vi "4.2.4.vi"() -> ()   [LabVIEW 2017]
panel:
  in  "stop":bool
  in  "Frequency 2":dbl
  in  "Frequency 1":dbl
  in  "Phase 2":dbl
  in  "Phase 1":dbl
  out "XY Graph":cluster{"X":dbl[], "Y":dbl[]}[](graph)
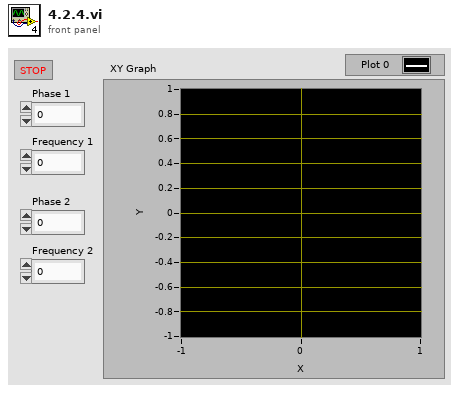
[diagram p1: front panel]
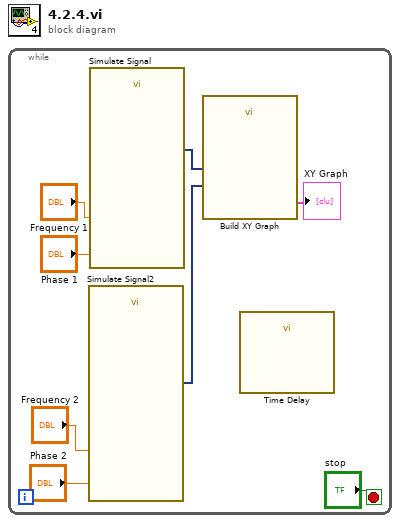
[diagram p0: block diagram]
diagram:
  n1 = while {
    stop <- "stop" stop-if-true
    n2 = call "Simulate Signal2"("Frequency"="Frequency 2", "Phase"="Phase 2") -> ("Sine"=w7:dynamicdata)  [unwired: 12 in, 1 out]
    n3 = call "Simulate Signal"("Frequency"="Frequency 1", "Phase"="Phase 1") -> ("Sine"=w8:dynamicdata)  [unwired: 12 in, 1 out]
    n4 = call "Build XY Graph"("Y Input"=w7, "X Input"=w8) -> ("XY Graph"=→"XY Graph":cluster{"X":dbl[], "Y":dbl[]}[])  [unwired: 8 in, 1 out]
    n5 = call "Time Delay"() -> ()  [unwired: 11 in, 1 out]
  }
